vi "ResonanceAnalyzer.vi"() -> ()   [LabVIEW 2015]
uses:
  <vilib>/imath/engines/lvmath2/RunTimeEngine/Managers/WorkSpace/UID Generator.vi
  <vilib>/imath/engines/lvmath2/RunTimeEngine/RangeToken/NIMS_Range.vi
  <instcachedir>/0/NIMS_Range_D919CC09935940E88F755EC1C6F49AC1.lvgen/NIMS_Range_D919CC09935940E88F755EC1C6F49AC1_000.vi
  <vilib>/imath/engines/lvmath2/RunTimeEngine/RunTimeType/NIMS_RunTimeType_From StrictType (excl LVString).vi
  <instcachedir>/0/NIMS_RunTimeType_From StrictType (excl LVString)_EB1C38A9BC5048DA9ABDA8F781E54D21.lvgen/NIMS_RunTimeType_From StrictType (excl LVString)_EB1C38A9BC5048DA9ABDA8F781E54D21_000.vi
  <vilib>/imathl/engines/lvmath/Functions/Error Handling/Create Error.vi
  <vilib>/imath/engines/lvmath2/RunTimeEngine/LocalVariableDefStatement/MC_LocalVariableDefStatement_Display.vi
  <vilib>/imath/engines/lvmath2/RunTimeEngine/BuiltInFunctions/size/NIMS_I32Row=size(GRow).vi
  <instcachedir>/0/NIMS_I32Row=size(GRow)_E5C05C6B13124B29B774CC4F993D3C59.lvgen/NIMS_I32Row=size(GRow)_E5C05C6B13124B29B774CC4F993D3C59_000.vi
  <vilib>/imath/engines/lvmath2/RunTimeEngine/ArithmeticOperatorToken/NIMS_ArithmeticOperator_minus.vi
  <instcachedir>/0/NIMS_ArithmeticOperator_minus_8228ED1EA52B4CB8A68367813E4B0C9D.lvgen/NIMS_ArithmeticOperator_minus_8228ED1EA52B4CB8A68367813E4B0C9D_003.vi
  <vilib>/imath/engines/lvmath2/RunTimeEngine/IndexRead/NIMS M(S,S).vi
  <instcachedir>/0/NIMS M(S,S)_AC51E74150A542F7991B9634C66F3096.lvgen/NIMS M(S,S)_AC51E74150A542F7991B9634C66F3096_002.vi
  <vilib>/imath/engines/lvmath2/RunTimeEngine/BuiltInFunctions/randnormal/NIMS_randnormal(1,I32).vi
  <vilib>/imath/engines/lvmath2/RunTimeEngine/ErrorHandling/NIMS_Error From Error Code.vi
  <vilib>/imath/engines/lvmath2/RunTimeEngine/ArithmeticOperatorToken/NIMS_ArithmeticOperator_plus.vi
  <instcachedir>/0/NIMS_ArithmeticOperator_plus_A4F2756F5ADB4A0090E0DBD7C10701C8.lvgen/NIMS_ArithmeticOperator_plus_A4F2756F5ADB4A0090E0DBD7C10701C8_005.vi
  <vilib>/imath/engines/lvmath2/RunTimeEngine/Managers/SymbolTable/Clear UID.vi
  <vilib>/imath/engines/lvmath2/RunTimeEngine/NodeEndStatement/NIMS_NodeEndStatement_Output.vi
  <instcachedir>/0/NIMS_NodeEndStatement_Output_53EC0D466D134D7ABD903AC30B43404B.lvgen/NIMS_NodeEndStatement_Output_53EC0D466D134D7ABD903AC30B43404B_005.vi
  <instcachedir>/0/NIMS_NodeEndStatement_Output_53EC0D466D134D7ABD903AC30B43404B.lvgen/NIMS_NodeEndStatement_Output_53EC0D466D134D7ABD903AC30B43404B_000.vi
  <vilib>/imath/engines/lvmath2/RunTimeEngine/ErrorHandling/NIMS_Finalize Error.vi
  <vilib>/Utility/file.llb/Read Delimited Spreadsheet (DBL).vi
  <vilib>/imath/engines/lvmath2/RunTimeEngine/Managers/SymbolTable/NIMS_WorkSpace.lvlib
panel:
  out "Resonance Curve":cluster{"all rows":dbl[], "all rows":dbl[]}[](graph)
  out "Results":T1={"Q"=0.8144410664899207, "Center Frequency"=464.2892632156428, "Amplitude"=0.18147113812722032}
  in  "Tab Control":enum32{"Simulation", "Experiment"}(tab)=enum."Experiment"
  in  "Input Parameters":T2={"Q"=10.0, "Center Frequency"=600.0, "Start Frequency"=400.0, "End Frequency"=800.0, "dF"=5.0, "Noise Level"=0.01}
  in  "File Path Control":path=path "C:/Users/mylicon/Desktop/week6/output-full"
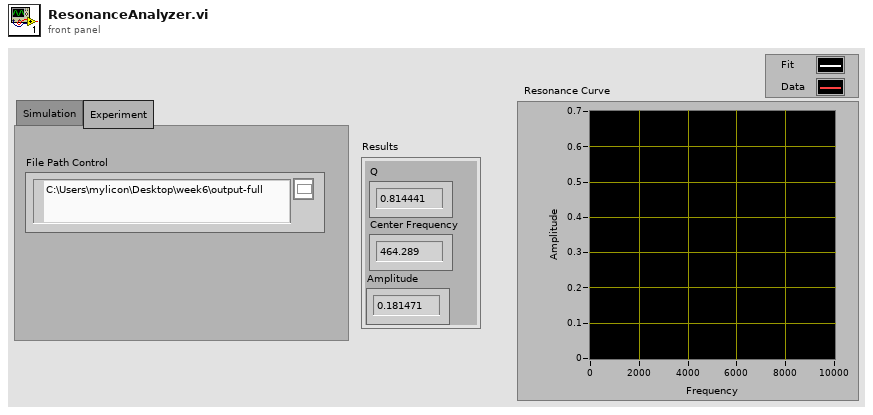
[diagram p1: front panel]
types:
  T1 = cluster{"Q":dbl, "Center Frequency":dbl, "Amplitude":dbl}
  T2 = cluster{"Q":dbl, "Center Frequency":dbl, "Start Frequency":dbl, "End Frequency":dbl, "dF":dbl, "Noise Level":dbl}
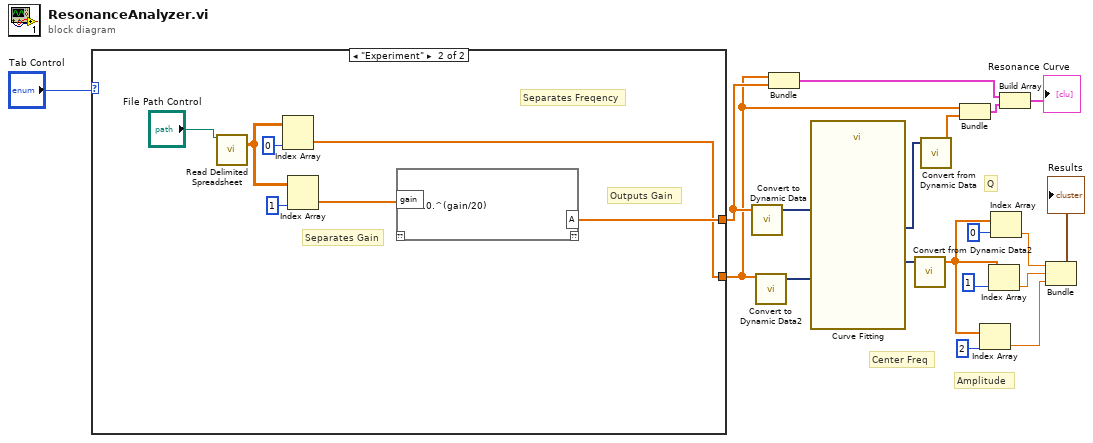
[diagram p0: block diagram]
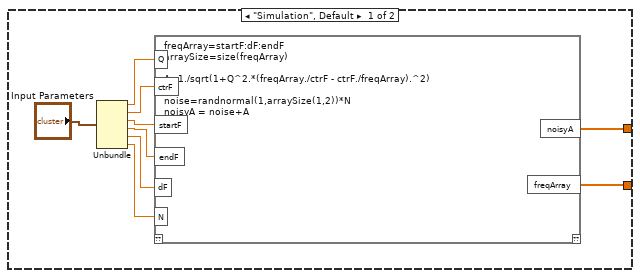
[diagram p2: hidden frame]
diagram:
  # "Center Freq"
  # "Amplitude"
  # "Q"
  n1 = case shown="\"Experiment\"" "Tab Control" {
    tunnel: [w21 w208] -> w2
    tunnel: [w20 w209] -> w3
    frame "Simulation", Default {
      n2 = Unbundle("Input Parameters") -> ("Q"=w26:dbl, "Center Frequency"=w25:dbl, "Start Frequency"=w22:dbl, "End Frequency"=w23:dbl, "dF"=w24:dbl, "Noise Level"=w27:dbl)
      n3 = mathscript code="freqArray=startF:dF:endF\narraySize=size(freqArray)\n\nA=1./sqrt(1+Q^2.*(freqArray./ctrF - ctrF./freqArray).^2)\n\nnoise=randnormal(1,arraySize(1,2))*N\nnoisyA = noise+A"("Q"=w26, "ctrF"=w25, "startF"=w22, "endF"=w23, "dF"=w24, "N"=w27) -> ("noisyA"=w20:cdb[], "freqArray"=w21:dbl[])  [unwired: 1 in, 1 out]
    }
    frame "Experiment" {
      # "Outputs Gain"
      # "Separates Freqency"
      # "Separates Gain"
      n4 = call-poly <vilib>:"Read Delimited Spreadsheet.vi"("file path (dialog if empty)"="File Path Control") -> ("all rows"=w212:dbl[][])  [unwired: 9 in, 5 out]
      n5 = Index Array(array=w212, index (col)=0 ("disabled index (col)")) -> (element=w208:dbl[])  [unwired: 1 in]
      n6 = Index Array(array=w212, index (col)=1 ("disabled index (col)")) -> (element=w210:dbl[])  [unwired: 1 in]
      n7 = mathscript code="A=10.^(gain/20)"("gain"=w210) -> ("A"=w209:dbl[])  [unwired: 1 in, 1 out]
    }
  }
  n8 = call "Convert to Dynamic Data"("Array"=w3) -> ("Dynamic Data Type"=w18:dynamicdata)  [unwired: 3 in]
  n9 = call "Convert to Dynamic Data2"("Array"=w2) -> ("Dynamic Data Type"=w4:dynamicdata)  [unwired: 3 in]
  n10 = Bundle("all rows"=w2, "noisyA"=w3) -> (w7:cluster{"all rows":dbl[], "noisyA":cdb[]})  [unwired: 1 in]
  n11 = call "Curve Fitting"("Locations"=w4, "Signals"=w18) -> ("best fit"=w17:dynamicdata, "non-linear coefficients"=w16:dynamicdata)  [unwired: 5 in, 3 out]
  n12 = call "Convert from Dynamic Data2"("Dynamic Data Type"=w16) -> ("Array"=w1:dbl[])  [unwired: 3 in]
  n13 = call "Convert from Dynamic Data"("Dynamic Data Type"=w17) -> ("Array"=w8:dbl[])  [unwired: 3 in]
  n14 = Bundle("all rows"=w2, "Array"=w8) -> (w6:cluster{"all rows":dbl[], "Array":dbl[]})  [unwired: 1 in]
  n15 = Index Array(array=w1, index=2) -> (element=w10:dbl)
  n16 = Index Array(array=w1, index=1) -> (element=w9:dbl)
  n17 = Index Array(array=w1, index=0) -> (element=w13:dbl)
  n18 = Build Array(w7, w6) -> (→"Resonance Curve":cluster{"all rows":dbl[], "noisyA":cdb[]}[])
  n19 = Bundle(w13, w9, w10) -> (→"Results":cluster{dbl, dbl, dbl})  [unwired: 1 in]
